vi "getIntrincZk.vi"(8 "error in (no error)":errorcluster, 9 "Field Idx":i32[](array[numeric]), 10 "Filter Type":T1, 11 "OptStateEsti in":refnum<class "OptStateEsti.lvclass">) -> (0 "error out":errorcluster, 2 "Intrinsic Zk":dbl[][](array[numeric]), 3 "OptStateEsti out":refnum<class "OptStateEsti.lvclass">)   [LabVIEW 2016, in "OptStateEsti.lvclass"]
doc: "Get the intrinsic zk of specific filter based on the array of field index. The output array shape is nx1."
uses:
  OptStateEsti.lvclass
  StrictDef/FilterType.ctl
  OptStateEsti.lvclass/OptStateEsti.ctl
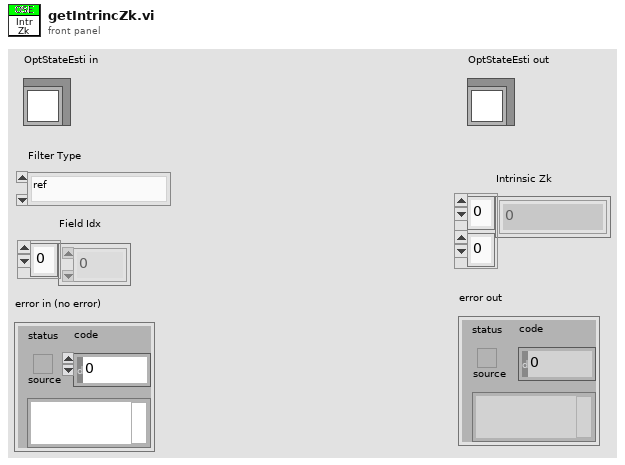
[diagram p1: front panel]
types:
  T1 = typedef "FilterType.ctl" = enum16{"ref", "u", "g", "r", "i", "z", "y"}
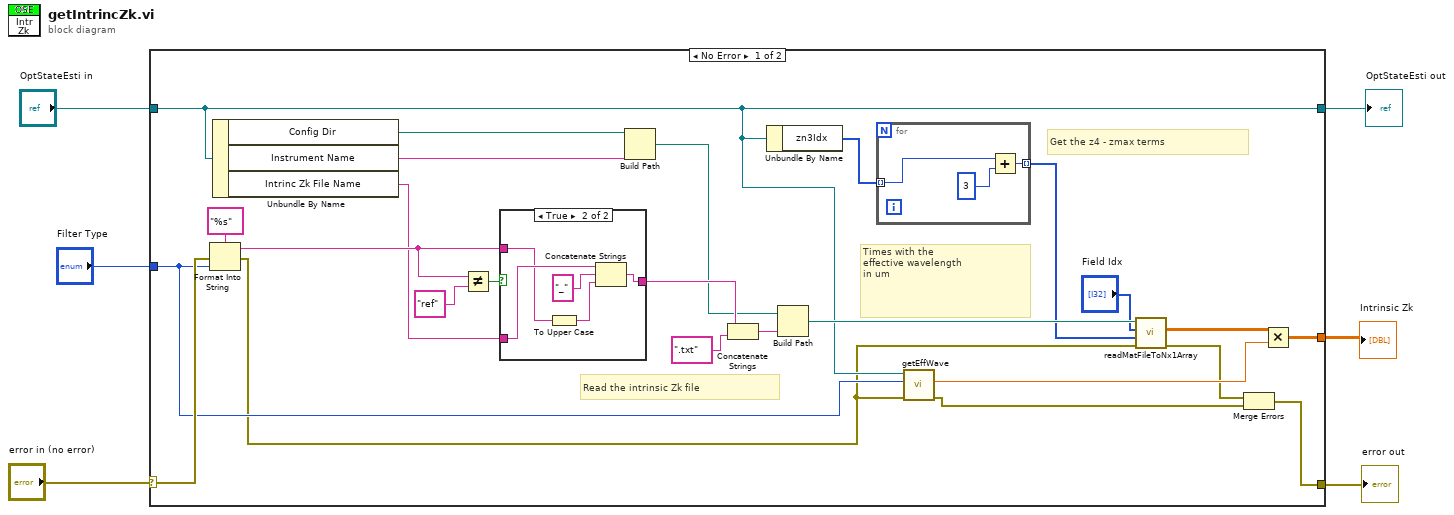
[diagram p0: block diagram]
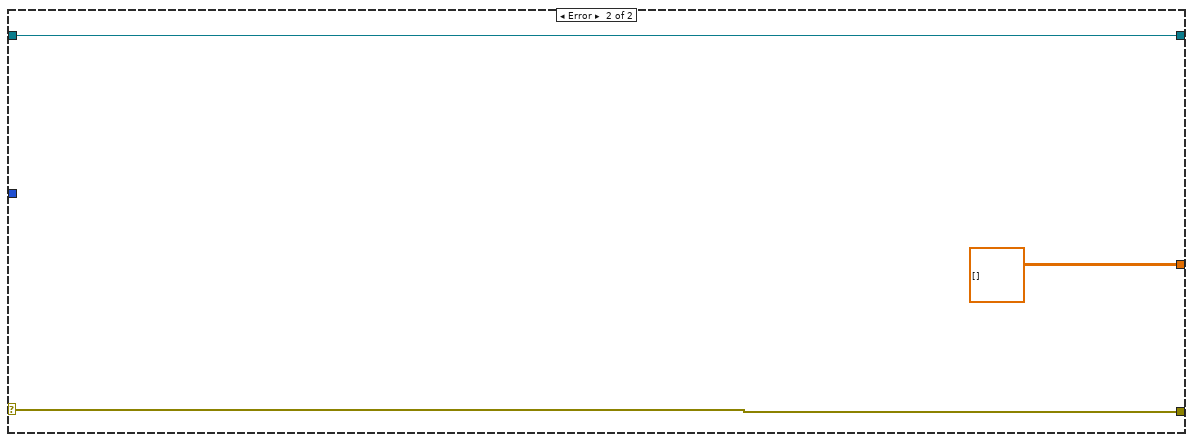
[diagram p3: hidden frame]
diagram:
  n1 = case shown="No Error" "error in (no error)" {
    selector: "error in (no error)" -> [w16 w43]
    tunnel: [w9 w43] -> w5
    tunnel: [w12 w42] -> w4
    tunnel: "OptStateEsti in" -> [w12 w42]
    tunnel: [w22 dbl[][] []] -> w3
    tunnel: "Filter Type" -> [w11 _]
    frame No Error {
      # "Times with the \neffective wavelength\nin um"
      # "Get the z4 - zmax terms"
      # "Read the intrinsic Zk file"
      n2 = Format Into String(format string="%s", error in=w16, w11) -> (resulting string=w15:string, error out=w10:errorcluster)  [unwired: 1 in]
      n3 = Unbundle By Name(w12) -> ("Config Dir"=w18:path, "Instrument Name"=w27:string, "Intrinc Zk File Name"=w14:string)
      n4 = Not Equal?(x=w15, y="ref") -> (x != y?=w31:bool)
      n5 = case shown="True" w31 {
        tunnel: w14 -> [w35 w40]
        tunnel: [w35 w36] -> w29
        tunnel: w15 -> [_ w38]
        frame False {
        }
        frame True {
          n6 = To Upper Case(1:w38) -> (0:w37:string)
          n7 = Concatenate Strings(w40, "_" ("string"), w37) -> (w36:string)
        }
      }
      n8 = Build Path(base path=w18, name or relative path=w27) -> (appended path=w26:path)
      n9 = Concatenate Strings(w29, ".txt" ("string")) -> (w25:string)
      n10 = Unbundle By Name(w12) -> ("zn3Idx"=w19:i32[])
      n11 = Build Path(base path=w26, name or relative path=w25) -> (appended path=w24:path)
      n12 = for {
        tunnel: w19 -> [w34] mode=indexing
        tunnel: [w33] -> w20 mode=indexing
        n13 = Add(x=w34, y=3) -> (x+y=w33:i32)
      }
      n14 = call "getEffWave.vi"("error in (no error)"=w10, "Filter Type"=w11, "OptStateEsti in"=w12) -> ("error out"=w7:errorcluster, "Effective Wavelength  (um)"=w13:dbl)  [unwired: 6 in, 1 out]
      n15 = call "readMatFileToNx1Array.vi"("error in (no error)"=w10, "Index of Column"=w20, "Index of Row"="Field Idx", "Path"=w24) -> ("error out"=w8:errorcluster, "nx1 Array"=w23:dbl[][])  [unwired: 6 in]
      n16 = Merge Errors(w8, w7) -> (w9:errorcluster)
      n17 = Multiply(x=w23, y=w13) -> (x*y=w22:dbl[][])
    }
    frame Error {
    }
  }
  "error out" <- w5
  "OptStateEsti out" <- w4
  "Intrinsic Zk" <- w3
